vi "Configure Trigger Model Recall Configuration List Block.vi"(0 "VISA resource name":refnum<visa-resource-name>, 1 "Block Number (1)":i32=1 format="%#.6g", 2 "Configuration List Name":string, 3 "Enable Index (False)":bool, 4 "Index (1)":i32=1 format="%#.6g", 5 "error in (no error)":errorcluster) -> (14 "VISA resource name out":refnum<visa-resource-name>, 19 "error out":errorcluster)   [LabVIEW 2020, in "Keithley 2450.lvlib"]
doc: "Recalls the system settings that are stored in a measure or source configuration list."
uses:
  Keithley 2450.lvlib
panel:
  # "False"
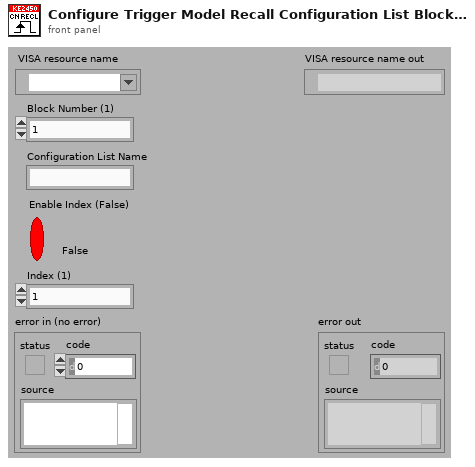
[diagram p1: front panel]
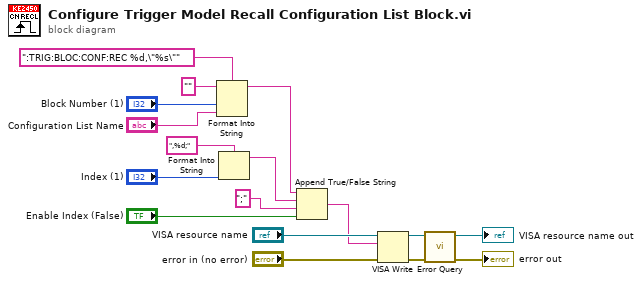
[diagram p0: block diagram]
diagram:
  n1 = Format Into String(format string=":TRIG:BLOC:CONF:REC %d,\"%s\"", initial string="", "Block Number (1)", "Configuration List Name") -> (resulting string=w4:string)  [unwired: 1 in, 1 out]
  n2 = Format Into String(format string=",%d;", "Index (1)") -> (resulting string=w2:string)  [unwired: 2 in, 1 out]
  n3 = Append True/False String(1:"Enable Index (False)", 2:";" ("true string"), 3:w2, 4:w4) -> (0:w3:string)
  n4 = VISA Write(VISA resource name="VISA resource name", write buffer=w3, error in (no error)="error in (no error)") -> (VISA resource name out=w13:refnum<visa-resource-name>, error out=w12:errorcluster)  [unwired: 1 out]
  n5 = call "Error Query.vi"("error in (no error)"=w12, "VISA resource name"=w13) -> ("error out"=→"error out":errorcluster, "VISA resource name out"=→"VISA resource name out":refnum<visa-resource-name>)  [unwired: 8 out]
